vi "Load Configuration Settings from XML.vi"(8 "error in (no error)":errorcluster caption="错误输入（无错误）", 11 "User Configuration in":T1={"Hardware Configuration"={"Physical Channel"="", "Maximum Input"=0.0, "Minimum Input"=0.0, "Sample Rate"=0.0, "Number of Samples"=0}, "Analysis Configuration"={"Statistics"=TRUE}, "New Data Behavior"=enum."Replace"} caption="用户配置输入") -> (0 "error out":errorcluster caption="错误输出", 3 "User Configuration out":T1={"Hardware Configuration"={"Physical Channel"="", "Maximum Input"=0.0, "Minimum Input"=0.0, "Sample Rate"=0.0, "Number of Samples"=0}, "Analysis Configuration"={"Statistics"=TRUE}, "New Data Behavior"=enum."Replace"} caption="用户配置输出")   [LabVIEW 2013]
doc: "尝试从XML文件加载先前的用户设置。\n\n该VI不会生成错误。如无法加载和解析XML文件，直接返回默认设置。"
uses:
  controls/User Specified Data.ctl
  controls/HW Configuration.ctl
  controls/Analysis Configuration.ctl
  controls/New Data Behavior.ctl
  <vilib>/Utility/xml.llb/Read From XML File(string).vi
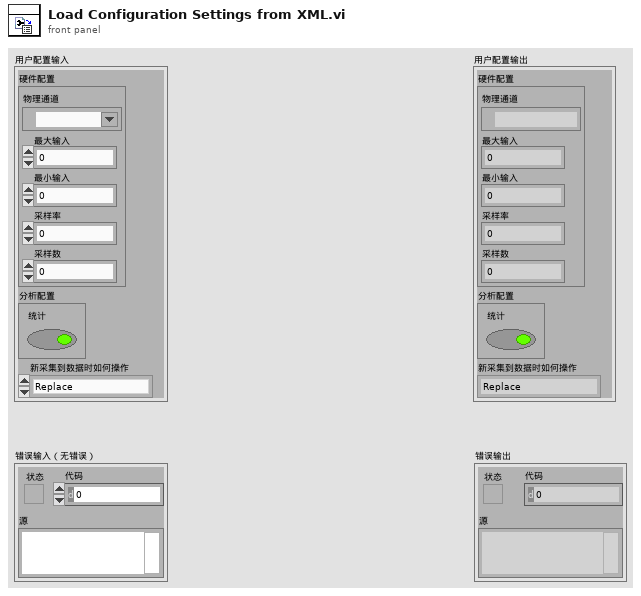
[diagram p1: front panel]
types:
  T1 = typedef "User Specified Data.ctl" = cluster{"Hardware Configuration":T2, "Analysis Configuration":T3, "New Data Behavior":T4}
  T2 = typedef "HW Configuration.ctl" = cluster{"Physical Channel":tag, "Maximum Input":dbl, "Minimum Input":dbl, "Sample Rate":dbl, "Number of Samples":i32}
  T3 = typedef "Analysis Configuration.ctl" = cluster{"Statistics":bool}
  T4 = typedef "New Data Behavior.ctl" = enum16{"Replace", "Overlay", "Append"}
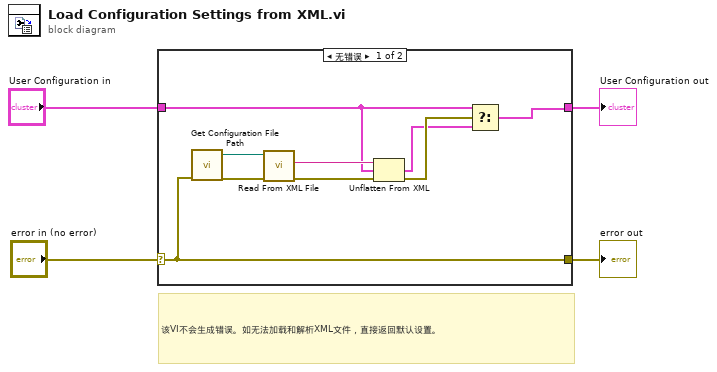
[diagram p0: block diagram]
diagram:
  # "该VI不会生成错误。如无法加载和解析XML文件，直接返回默认设置。"
  n1 = case shown="无错误" "error in (no error)" {
    selector: "error in (no error)" -> [w10 w15]
    tunnel: [w10 w15] -> w3
    tunnel: "User Configuration in" -> [w7 w14]
    tunnel: [w5 w14] -> w1
    frame No Error {
      n2 = call "Get Configuration File Path.vi"("error in (no error)"=w10) -> ("error out"=w12:errorcluster, "XML File Path"=w13:path)  [unwired: 9 in]
      n3 = call-poly <vilib>:"Read From XML File.vi"("error in (no error)"=w12, "XML File Path"=w13) -> ("error out"=w9:errorcluster, "XML Elements"=w11:string)  [unwired: 7 in, 1 out]
      n4 = Unflatten From XML(xml string=w11, type=w7, error in (no error)=w9) -> (value=w6:T1, error out=w8:errorcluster)
      n5 = Select(t=w7, s=w8, f=w6) -> (s? t:f=w5:T1)
    }
    frame Error {
    }
  }
  "error out" <- w3
  "User Configuration out" <- w1
